vi "Magna Power Scan.vi"(8 "error in (no error)":errorcluster, 10 "Magna Power.lvclass":refnum<class "Magna Power.lvclass">, 11 "Magna Power Scan.lvclass in":refnum<class "Magna Power Scan.lvclass">) -> (0 "error out":errorcluster, 3 "Magna Power Scan.lvclass out":refnum<class "Magna Power Scan.lvclass">)   [LabVIEW 2012, in "Magna Power Scan.lvclass"]
uses:
  Magna Power Scan.lvclass
  Instruments/Magna-Power Power Supply/Magna Power.lvclass
  Scanner/Scanner.lvclass
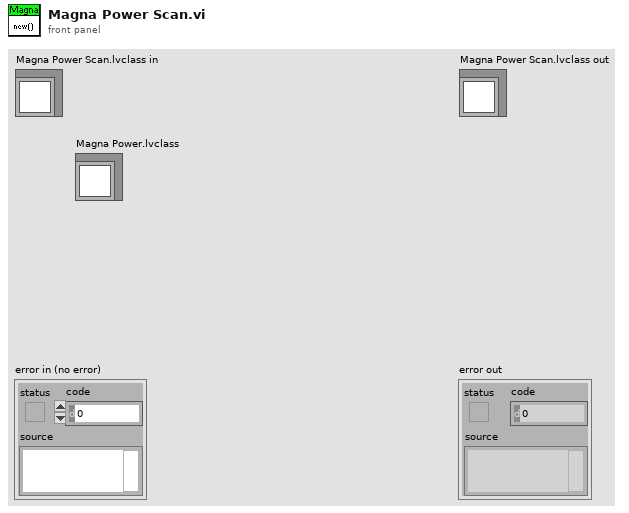
[diagram p1: front panel]
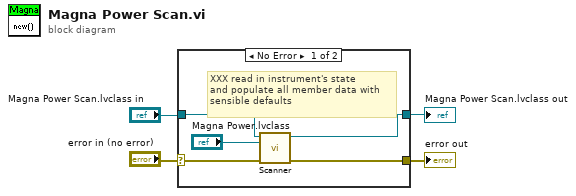
[diagram p0: block diagram]
diagram:
  n1 = case shown="No Error" "error in (no error)" {
    selector: "error in (no error)" -> [w9 w11]
    tunnel: [w7 w11] -> w1
    tunnel: [w6 w10] -> w3
    tunnel: "Magna Power Scan.lvclass in" -> [w8 w10]
    frame No Error {
      # "XXX read in instrument's state\nand populate all member data with\nsensible defaults"
      n2 = call "Scanner.vi"("error in (no error)"=w9, "Scannable"="Magna Power.lvclass", "Scanner.lvclass in"=w8) -> ("error out"=w7:errorcluster, "Scanner.lvclass out"=w6:refnum<class "Magna Power Scan.lvclass">)  [unwired: 1 in, 6 out]
    }
    frame Error {
    }
  }
  "error out" <- w1
  "Magna Power Scan.lvclass out" <- w3
